vi "GenerateArmMotionProfilePoints.vi"(4 "MotionProfileGeneratorParameters":T4={"Trajectory Point Interval (ms)"=10, "Maximum Travel Speed (units/s)"=0.0, "Velocity Ramp Time (ms)"=0.0, "Acceleration Ramp Time (ms)"=1.0} {"Acceleration Ramp Time (ms)" min=1.0; "Velocity Ramp Time (ms)" min=1.0; "Maximum Travel Speed (units/s)" min=0.0; "Trajectory Point Interval (ms)" items=["TrajectoryDuration_0ms"=0, "TrajectoryDuration_5ms"=5, "TrajectoryDuration_10ms"=10, "TrajectoryDuration_20ms"=20, "TrajectoryDuration_30ms"=30, "TrajectoryDuration_40ms"=40, "TrajectoryDuration_50ms"=50, "TrajectoryDuration_100ms"=100]}, 5 "PathDistance":dbl, 6 "ArmPathIn":T3[](array[typedef]), 7 "IndexedPathLength":dbl[](array[numeric])) -> (0 "ArmPathOut":T3[](array[typedef]), 1 "WristPath":T1[](array[typedef]) {"Time (ms)" items=["TrajectoryDuration_0ms"=0, "TrajectoryDuration_5ms"=5, "TrajectoryDuration_10ms"=10, "TrajectoryDuration_20ms"=20, "TrajectoryDuration_30ms"=30, "TrajectoryDuration_40ms"=40, "TrajectoryDuration_50ms"=50, "TrajectoryDuration_100ms"=100]}, 2 "ExtendPath":T1[](array[typedef]) {"Time (ms)" items=["TrajectoryDuration_0ms"=0, "TrajectoryDuration_5ms"=5, "TrajectoryDuration_10ms"=10, "TrajectoryDuration_20ms"=20, "TrajectoryDuration_30ms"=30, "TrajectoryDuration_40ms"=40, "TrajectoryDuration_50ms"=50, "TrajectoryDuration_100ms"=100]}, 3 "ShoulderPath":T1[](array[typedef]) {"Time (ms)" items=["TrajectoryDuration_0ms"=0, "TrajectoryDuration_5ms"=5, "TrajectoryDuration_10ms"=10, "TrajectoryDuration_20ms"=20, "TrajectoryDuration_30ms"=30, "TrajectoryDuration_40ms"=40, "TrajectoryDuration_50ms"=50, "TrajectoryDuration_100ms"=100]})   [LabVIEW 2018]
uses:
  TypeDefs/ArmCoordinate.ctl
  General/MotionProfiling/TypeDefs/MotionProfileGeneratorParams.ctl
  <vilib>/Rock Robotics/WPI/ThirdParty/Phoenix-LabVIEW/Motor Controller/Controls/CTRE_Phoenix_MotorControl_TrajectoryPointTimeDur.ctl
  General/MotionProfiling/TypeDefs/TrajectoryPoint.ctl
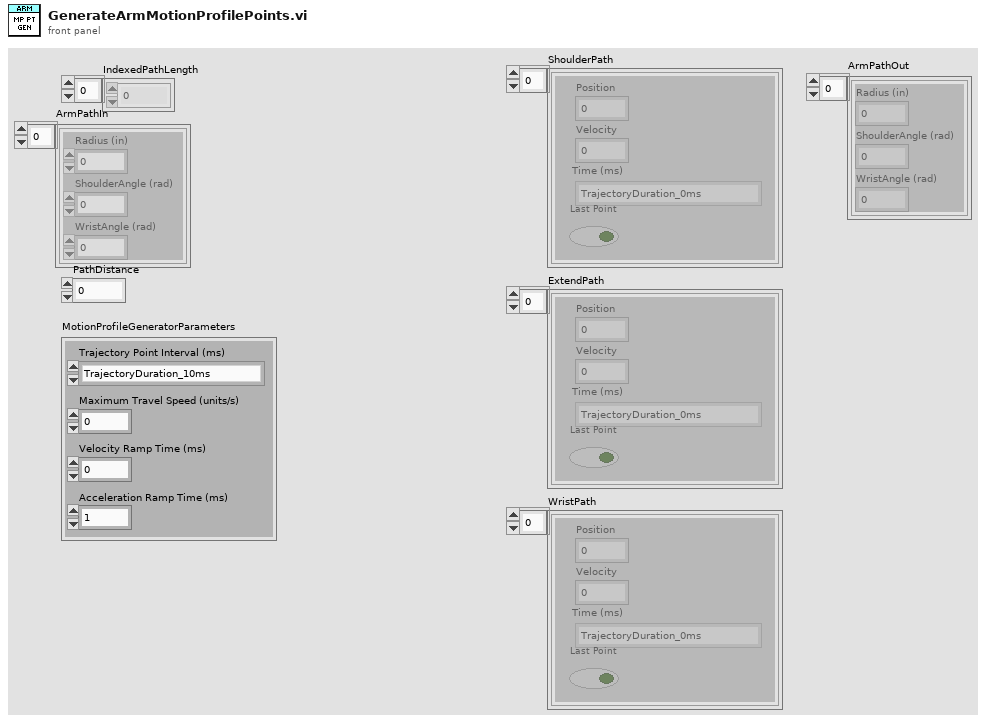
[diagram p1: front panel]
types:
  T1 = typedef "TrajectoryPoint.ctl" = cluster{"Position ":dbl, "Velocity ":dbl, "Time (ms)":T2, "Last Point":bool}
  T2 = typedef "CTRE_Phoenix_MotorControl_TrajectoryPointTimeDur.ctl" = i32
  T3 = typedef "ArmCoordinate.ctl" = cluster{"Radius (in)":dbl, "ShoulderAngle (rad)":dbl, "WristAngle (rad)":dbl}
  T4 = typedef "MotionProfileGeneratorParams.ctl" = cluster{"Trajectory Point Interval (ms)":T2, "Maximum Travel Speed (units/s)":dbl, "Velocity Ramp Time (ms)":dbl, "Acceleration Ramp Time (ms)":dbl}
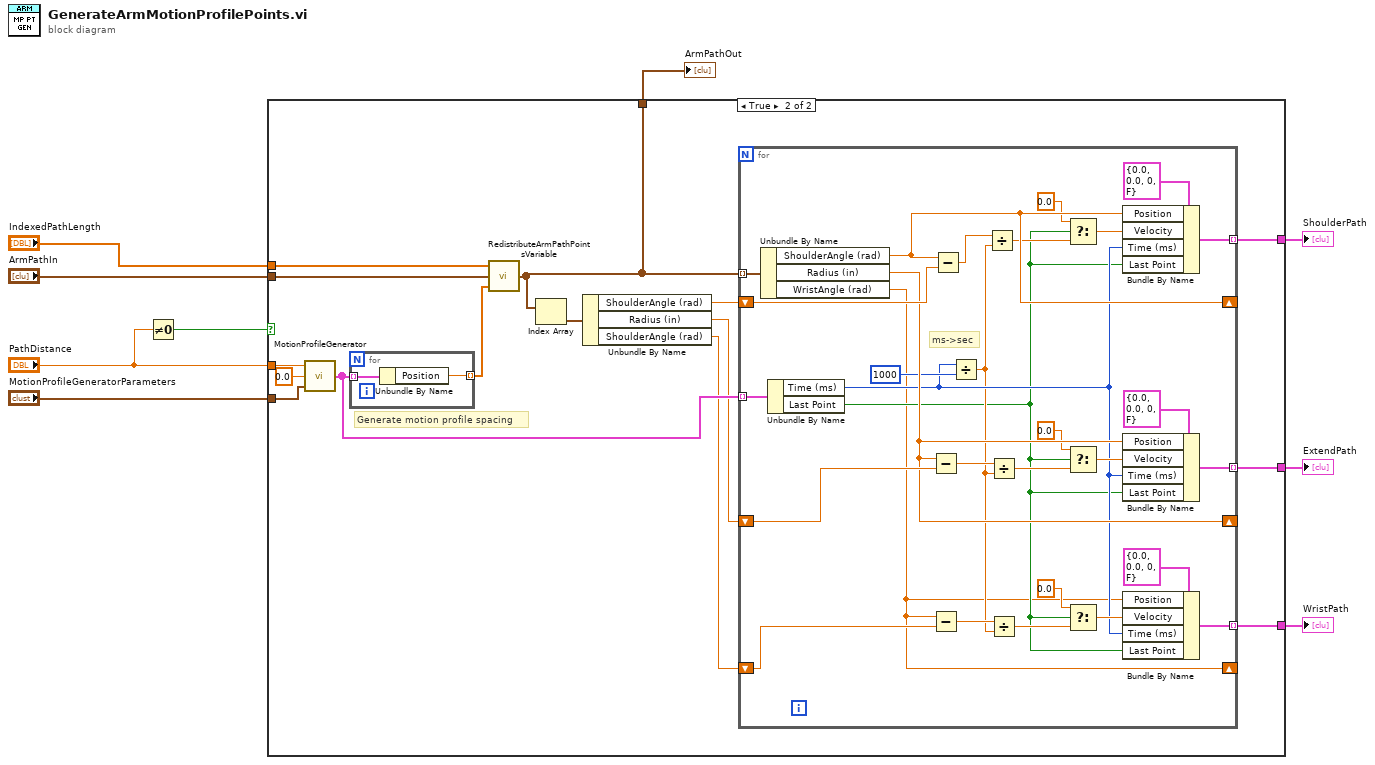
[diagram p0: block diagram]
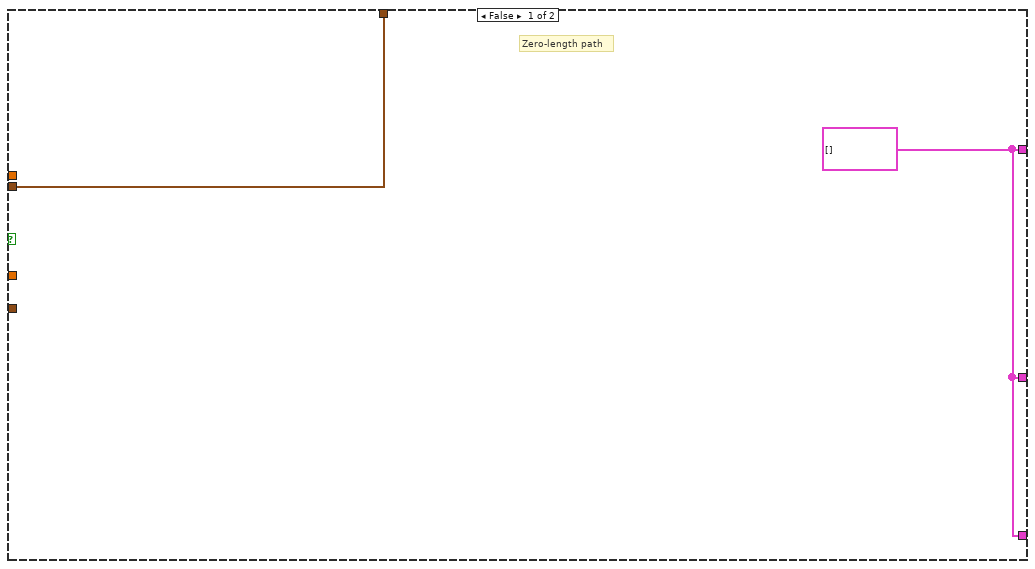
[diagram p2: hidden frame]
diagram:
  n1 = Not Equal To 0?(x="PathDistance") -> (x != 0?=w2:bool)
  n2 = case shown="True" w2 {
    tunnel: "ArmPathIn" -> [w11 w24]
    tunnel: "IndexedPathLength" -> [_ w23]
    tunnel: "MotionProfileGeneratorParameters" -> [_ w22]
    tunnel: [w10 w21] -> w6
    tunnel: [w10 w20] -> w5
    tunnel: "PathDistance" -> [_ w15]
    tunnel: [w11 w14] -> w3
    tunnel: [w10 w12] -> w1
    frame False {
      w10 = T1[] []
      # "Zero-length path"
    }
    frame True {
      # "Generate motion profile spacing"
      n3 = call "MotionProfileGenerator.vi"("MotionProfileGeneratorParameters"=w22, "Starting Position (units)"=0.0 ("Starting Position (rotations)"), "Travel Distance (units)"=w15) -> ("Trajectory Points"=w18:T1[])
      n4 = for {
        tunnel: w18 -> [w58] mode=indexing
        tunnel: [w57] -> w25 mode=indexing
        n5 = Unbundle By Name(w58) -> ("Position"=w57:dbl)
      }
      n6 = call "RedistributeArmPathPointsVariable.vi"("DesiredPointSpacing"=w25, "ArmPathIn"=w24, "IndexedPathLength"=w23) -> ("ArmPathOut"=w14:T3[])
      n7 = Index Array(array=w14) -> (element=w19:T3)  [unwired: 1 in]
      n8 = Unbundle By Name(w19) -> ("ShoulderAngle (rad)"=w17:dbl, "Radius (in)"=w16:dbl, "ShoulderAngle (rad)"=w13:dbl)
      n9 = for {
        tunnel: w14 -> [w51] mode=indexing
        tunnel: w18 -> [w52] mode=indexing
        tunnel: [w54] -> w20 mode=indexing
        tunnel: [w53] -> w21 mode=indexing
        shift-right: [w49] -> _
        shift-left: w17 -> [w50]
        shift-right: [w47] -> _
        shift-left: w16 -> [w48]
        shift-right: [w28] -> _
        shift-left: w13 -> [w31]
        tunnel: [w27] -> w12 mode=indexing
        # "ms->sec"
        n10 = Unbundle By Name(w51) -> ("ShoulderAngle (rad)"=w49:dbl, "Radius (in)"=w47:dbl, "WristAngle (rad)"=w28:dbl)
        n11 = Unbundle By Name(w52) -> ("Time (ms)"=w32:T2, "Last Point"=w29:bool)
        n12 = Subtract(x=w47, y=w48) -> (x-y=w46:dbl)
        n13 = Subtract(x=w28, y=w31) -> (x-y=w34:dbl)
        n14 = Subtract(x=w49, y=w50) -> (x-y=w45:dbl)
        n15 = Divide(x=w32, y=1000) -> (x/y=w30:dbl)
        n16 = Divide(x=w45, y=w30) -> (x/y=w44:dbl)
        n17 = Divide(x=w46, y=w30) -> (x/y=w41:dbl)
        n18 = Divide(x=w34, y=w30) -> (x/y=w35:dbl)
        n19 = Select(t=0.0, s=w29, f=w44) -> (s? t:f=w43:dbl)
        n20 = Select(t=0.0, s=w29, f=w41) -> (s? t:f=w40:dbl)
        n21 = Select(t=0.0, s=w29, f=w35) -> (s? t:f=w36:dbl)
        n22 = Bundle By Name(cluster=T1 {"Position "=0.0, "Velocity "=0.0, "Time (ms)"=0, "Last Point"=FALSE} ("trajectory point"), "Position"=w49, "Velocity"=w43, "Time (ms)"=w32, "Last Point"=w29) -> (w53:T1)
        n23 = Bundle By Name(cluster=T1 {"Position "=0.0, "Velocity "=0.0, "Time (ms)"=0, "Last Point"=FALSE} ("trajectory point"), "Position"=w47, "Velocity"=w40, "Time (ms)"=w32, "Last Point"=w29) -> (w54:T1)
        n24 = Bundle By Name(cluster=T1 {"Position "=0.0, "Velocity "=0.0, "Time (ms)"=0, "Last Point"=FALSE} ("trajectory point"), "Position"=w28, "Velocity"=w36, "Time (ms)"=w32, "Last Point"=w29) -> (w27:T1)
      }
    }
  }
  "ShoulderPath" <- w6
  "ExtendPath" <- w5
  "ArmPathOut" <- w3
  "WristPath" <- w1
